vi "Core.vi"(8 "error in (no error)":errorcluster, 10 "Actor in":refnum<class "Actor.lvclass">, 11 "Timed Msg in":refnum<class "Timed Msg.lvclass">) -> (0 "error out":errorcluster, 1 "Data":refnum<class "Data.lvclass">, 2 "Actor out":refnum<class "Actor.lvclass">, 3 "Timed Msg out":refnum<class "Timed Msg.lvclass">)   [LabVIEW 2020, in "Publisher.lvlib" / "Timed Msg.lvclass"]
doc: "Core of the Reponse Msg. Put the active code here.\n\nThis implementation does nothing."
uses:
  Timed Msg.lvclass
  PPL/HDH.Data.Generic.lvlibp/Data.lvclass
  PPL/HDH.Actor Framework.Core.Actor.lvlibp/1abvi3w/vi.lib/ActorFramework/Actor/Actor.lvclass
  Response Msg/Response Msg.lvclass
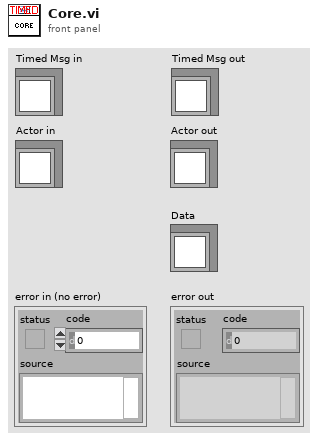
[diagram p1: front panel]
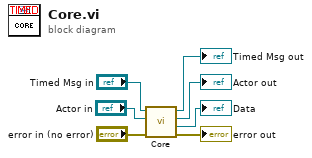
[diagram p0: block diagram]
diagram:
  n1 = call-parent "Core.vi"("error in (no error)"="error in (no error)", "Actor in"="Actor in", "Response Msg in"="Timed Msg in") -> ("error out"=→"error out":errorcluster, "Data"=→"Data":refnum<class "Data.lvclass">, "Actor out"=→"Actor out":refnum<class "Actor.lvclass">, "Response Msg out"=→"Timed Msg out":refnum<class "Timed Msg.lvclass">)  [unwired: 5 in]
